vi "Pressure Max Read Single.vi"(8 "error in":errorcluster, 9 "Channel Index":i32=1, 11 "Chiller in":refnum<class "Chiller.lvclass">) -> (0 "error out":errorcluster, 1 "Changed or First Call?":bool, 2 "Pressure Max SP":dbl, 3 "Chiller out":refnum<class "Chiller.lvclass">)   [LabVIEW 2023, in "Chiller.lvclass"]
uses:
  Chiller.lvclass
  Chiller.lvclass/Chiller.ctl
  Low Level Capabilities/Pressure/Pressure Limit/Pressure Limit.lvclass
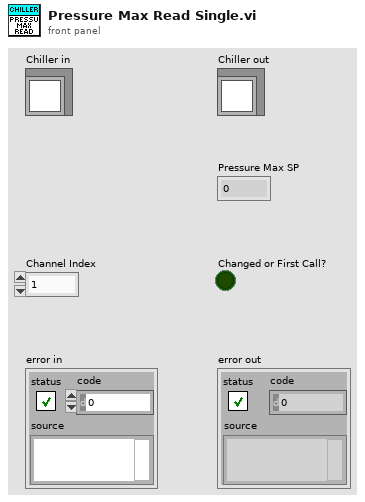
[diagram p1: front panel]
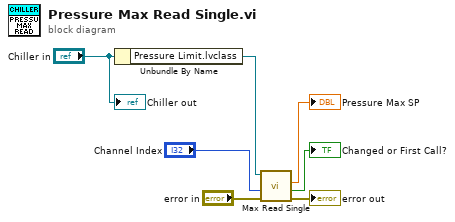
[diagram p0: block diagram]
diagram:
  n1 = Unbundle By Name("Chiller in") -> ("Pressure Limit.lvclass"=w7:refnum<class "Pressure Limit.lvclass">)
  n2 = call-dynamic "Max Read Single.vi"("error in"="error in", "Channel Index"="Channel Index", "Max Pressure Limit in"=w7) -> ("error out"=→"error out":errorcluster, "Changed or First Call?"=→"Changed or First Call?":bool, "Pressure Max SP"=→"Pressure Max SP":dbl)  [unwired: 5 in, 1 out]
  "Chiller out" <- "Chiller in"
